vi "Launch Syringe Heater.vi"(8 "error in (no error)":errorcluster, 11 "cRIO-CO2 in":refnum<class "cRIO-CO2.lvclass">) -> (0 "error out":errorcluster, 3 "cRIO-CO2 out":refnum<class "cRIO-CO2.lvclass">)   [LabVIEW 2015, in "cRIO-Carbondioxide.lvlib" / "cRIO-CO2.lvlib" / "cRIO-CO2.lvclass"]
uses:
  cRIO-CO2.lvclass
  Freezers Enumerator.ctl
  cRIO-CO2.lvclass/cRIO-CO2.ctl
  cRIO-CO2 Messages/Log Message Msg/Log Message Msg.lvclass/Log Message Msg.ctl
  <vilib>/ActorFramework/Message Enqueuer/Message Enqueuer.lvclass/Message Enqueuer.ctl
  <vilib>/ActorFramework/Message Enqueuer/Enqueue.vi
  <vilib>/ActorFramework/Message Priority Queue/Priority Enqueue.vi
  cRIO-CO2 Messages/Log Message Msg/Log Message Msg.lvclass
  <vilib>/ActorFramework/Message Enqueuer/Message Enqueuer.lvclass
  Heater/Heater.lvclass
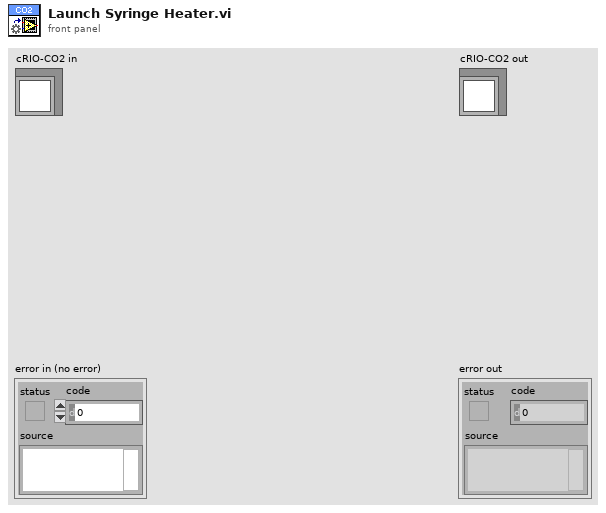
[diagram p1: front panel]
types:
  T1 = cluster{"Heater Duty Cycle SHV":refnum<k21>, "Thermocouple SHV":refnum<k21>, "Setpoint SHV":refnum<k21>, "Switch SHV":refnum<k21>}
  T2 = typedef "cRIO-Carbondioxide.lvlib/cRIO-CO2.lvlib/cRIO-CO2.lvclass/Freezers Enumerator.ctl" = enum16{"Undefined", "Syringe", "Cold Tank 1", "Cold Tank 2", "Cold Tank 3", "Cold Tank 4"}
  T3 = cluster{"PID":cluster{"P":dbl, "I":dbl, "D":dbl}, "Upper Limit":dbl, "Lower Limit":dbl}
  T4 = typedef "Dedicated Enqueuers.ctl" = cluster{"Freezers":cluster{"Syringe":refnum<class "Message Enqueuer.lvclass">, "Tank 1":refnum<class "Message Enqueuer.lvclass">, "Tank 2":refnum<class "Message Enqueuer.lvclass">, "Tank 3":refnum<class "Message Enqueuer.lvclass">, "Tank 4":refnum<class "Message Enqueuer.lvclass">}, "Heaters":cluster{"Syringe":refnum<class "Message Enqueuer.lvclass">, "Piston":refnum<class "Message Enqueuer.lvclass">}, "Blowers":cluster{"Tank 1":refnum<class "Message Enqueuer.lvclass">, "Tank 2":refnum<class "Message Enqueuer.lvclass">, "Tank 3":refnum<class "Message Enqueuer.lvclass">, "Tank 4":refnum<class "Message Enqueuer.lvclass">, "Syringe":refnum<class "Message Enqueuer.lvclass">}, "Sample Line":refnum<class "Message Enqueuer.lvclass">, "Storage Line":refnum<class "Message Enqueuer.lvclass">, "Transfer Line":refnum<class "Message Enqueuer.lvclass">, "Syringe Stepper":refnum<class "Message Enqueuer.lvclass">, "Syringe Line":refnum<class "Message Enqueuer.lvclass">, "Capillary Line":refnum<class "Message Enqueuer.lvclass">, "Preparation Line":refnum<class "Message Enqueuer.lvclass">, "Turbo":refnum<class "Message Enqueuer.lvclass">, "Vacuum":refnum<class "Message Enqueuer.lvclass">, "He Line":refnum<class "Message Enqueuer.lvclass">, "Cylinder":refnum<class "Message Enqueuer.lvclass">}
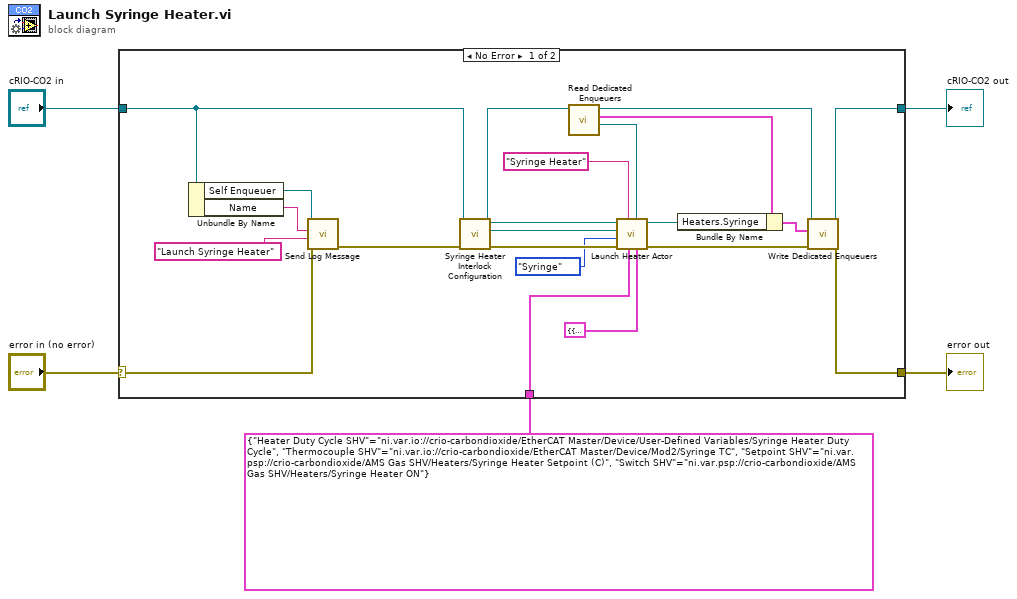
[diagram p0: block diagram]
diagram:
  n1 = case shown="No Error" "error in (no error)" {
    selector: "error in (no error)" -> [w23 w28]
    tunnel: [w15 w28] -> w4
    tunnel: [w16 w27] -> w2
    tunnel: "cRIO-CO2 in" -> [w17 w27]
    tunnel: T1 {"Heater Duty Cycle SHV"="ni.var.io://crio-carbondioxide/EtherCAT Master/Device/User-Defined Variables/Syringe Heater Duty Cycle", "Thermocouple SHV"="ni.var.io://crio-carbondioxide/EtherCAT Master/Device/Mod2/Syringe TC", "Setpoint SHV"="ni.var.psp://crio-carbondioxide/AMS Gas SHV/Heaters/Syringe Heater Setpoint (C)", "Switch SHV"="ni.var.psp://crio-carbondioxide/AMS Gas SHV/Heaters/Syringe Heater ON"} -> [w21 _]
    frame No Error {
      n2 = Unbundle By Name(w17) -> ("Self Enqueuer"=w22:refnum<class "Message Enqueuer.lvclass">, "Name"=w25:string)
      n3 = call "Send Log Message.vi"("error in (no error)"=w23, "String"="Launch Syringe Heater", "Source Name"=w25, "Message Enqueuer"=w22) -> ("error out"=w20:errorcluster)  [unwired: 6 in, 1 out]
      n4 = call "Syringe Heater Interlock Configuration.vi"("error in (no error)"=w20, "cRIO-CO2 in"=w17) -> ("error out"=w19:errorcluster, "Interlock Chain"=w18:refnum<class "Interlock Chain.lvclass">, "cRIO-CO2 out"=w12:refnum<class "cRIO-CO2.lvclass">)  [unwired: 7 in]
      n5 = call "Read Dedicated Enqueuers.vi"("cRIO-CO2 in"=w12) -> ("Qs.DedicatedEnQrs"=w8:refnum<queue>, "Dedicated Enqueuers"=w14:T4, "cRIO-CO2 out"=w7:refnum<class "cRIO-CO2.lvclass">)  [unwired: 7 in, 1 out]
      n6 = call "Launch Heater Actor.vi"("PID."=T3 {"PID"={"P"=200.0, "I"=4.0, "D"=100.0}, "Upper Limit"=200.0, "Lower Limit"=-100.0}, "DedicatedEnQrs"=w8, "SHVs"=w21, "Name"="Syringe Heater", "error in (no error)"=w19, "Freezer"=Freezers_Enumerator."Syringe", "Interlock Chain"=w18, "Caller Actor in"=w12) -> ("error out"=w9:errorcluster, "Caller-To-Actor Enqueuer"=w13:refnum<class "Message Enqueuer.lvclass">)  [unwired: 2 in]
      n7 = Bundle By Name(cluster=w14, "Heaters.Syringe"=w13) -> (w6:T4)
      n8 = call "Write Dedicated Enqueuers.vi"("error in (no error)"=w9, "Dedicated Enqueuers"=w6, "cRIO-CO2 in"=w7) -> ("error out"=w15:errorcluster, "cRIO-CO2 out"=w16:refnum<class "cRIO-CO2.lvclass">)  [unwired: 7 in]
    }
    frame Error {
    }
  }
  "error out" <- w4
  "cRIO-CO2 out" <- w2
